vi "Request Data JSON.vi"(8 "error in (no error)":errorcluster, 11 "GetSceneItemEnabled in":refnum<class "GetSceneItemEnabled.lvclass">) -> (0 "error out":errorcluster, 2 "Request Data JSON":string, 3 "GetSceneItemEnabled out":refnum<class "GetSceneItemEnabled.lvclass">)   [LabVIEW 2022 SP3, in "obs-websocket-lv.lvlib" / "GetSceneItemEnabled.lvclass"]
uses:
  GetSceneItemEnabled.lvclass
  GetSceneItemEnabled.lvclass/GetSceneItemEnabled.ctl
  <vilib>/IlluminatedG/lv-web-crypto/lv-json/JSON/JSON.lvlib
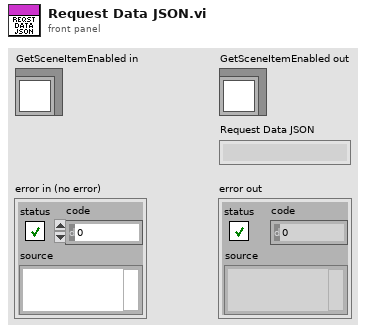
[diagram p1: front panel]
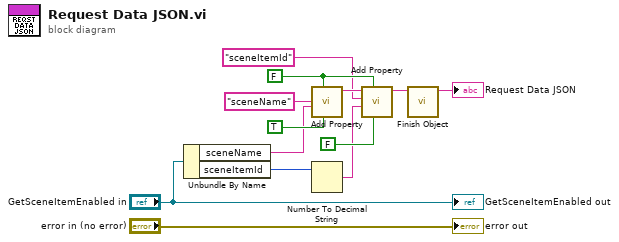
[diagram p0: block diagram]
diagram:
  w6 = FALSE ("Include Empty?")
  n1 = Unbundle By Name("GetSceneItemEnabled in") -> ("sceneName"=w9:string, "sceneItemId"=w11:i32)
  n2 = call <vilib>:"Add Property.vi"("String?"=TRUE, "Include Empty?"=w6, "Value"=w9, "Property Name"="sceneName") -> ("String out"=w7:string)  [unwired: 7 in]
  n3 = Number To Decimal String(number=w11) -> (decimal integer string=w3:string)  [unwired: 1 in]
  n4 = call <vilib>:"Add Property.vi"("String?"=FALSE, "Include Empty?"=w6, "Value"=w3, "Property Name"="sceneItemId", "String In"=w7) -> ("String out"=w2:string)  [unwired: 6 in]
  n5 = call <vilib>:"Finish Object.vi"("String In"=w2) -> ("String out"=→"Request Data JSON":string)  [unwired: 10 in]
  "error out" <- "error in (no error)"
  "GetSceneItemEnabled out" <- "GetSceneItemEnabled in"
